vi "ILL_ON-OFF.vi"(8 "error in (no error)":errorcluster, 10 "Boolean":bool, 11 "channel":refnum<k24>) -> (0 "error out":errorcluster)   [LabVIEW 2021]
uses:
  F:/2PhotonVision/psychometric_function_v2/lib/Grpc.Core.dll
  lib/Grpc.Core.dll
  F:/2PhotonVision/psychometric_function_v2/lib/FossilProtosSharp.dll
  lib/FossilProtosSharp.dll
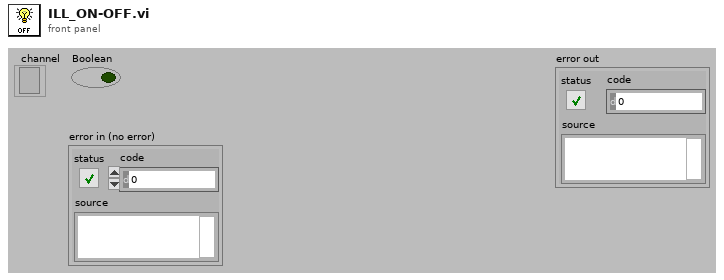
[diagram p1: front panel]
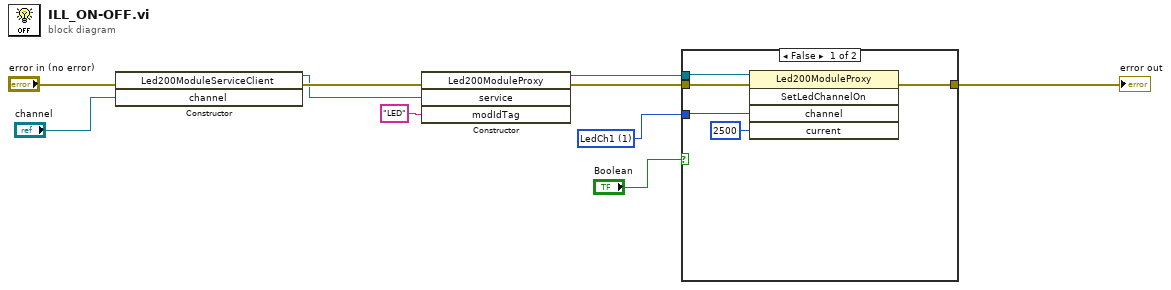
[diagram p0: block diagram]
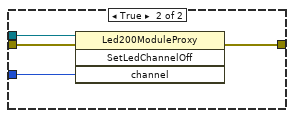
[diagram p2: hidden frame]
diagram:
  w10 = 1 items=["LedChUnspecified", "LedCh1", "LedCh2", "LedCh3", "LedCh4"] ("channel")
  n1 = constructor class="Led200ModuleServiceClient"(error in="error in (no error)", "channel"="channel") -> (reference out=w3:refnum<k24>, error out=w5:errorcluster)  [unwired: 2 in, 2 out]
  n2 = constructor class="Led200ModuleProxy"(error in=w5, "service"=w3, "modIdTag"="LED") -> (reference out=w7:refnum<k24>, error out=w8:errorcluster)  [unwired: 2 in, 3 out]
  n3 = case shown="False" "Boolean" {
    tunnel: w10 -> [w15 w19]
    tunnel: w8 -> [w13 w18]
    tunnel: w7 -> [w12 w17]
    tunnel: [w11 w16] -> w1
    frame False {
      n4 = invoke class="Led200ModuleProxy" method="SetLedChannelOn"(reference=w12, error in=w13, "channel"=w15, "current"=2500) -> (error out=w11:errorcluster)  [unwired: 1 in, 4 out]
    }
    frame True {
      n5 = invoke class="Led200ModuleProxy" method="SetLedChannelOff"(reference=w17, error in=w18, "channel"=w19) -> (error out=w16:errorcluster)  [unwired: 1 in, 3 out]
    }
  }
  "error out" <- w1
